vi "niDTS WLAN UTIL to Type.vi"(4 "N_SS":i32=1, 6 "MCS":i32, 9 "OFDM Data Rate (Mbps)":T1, 10 "DSSS Data Rate (Mbps)":T2, 11 "Standard":T3 caption="802.11 Standard") -> (2 "WLAN Type":T4)   [LabVIEW 2015, in "niDTS WLAN.lvlib"]
uses:
  niDTS WLAN.lvlib
  Includes/niDTS WLAN INC Type.ctl
  Includes/niDTS WLAN INC Standard.ctl
  Includes/niDTS WLAN INC DSSS Data Rate.ctl
  Includes/niDTS WLAN INC OFDM Data Rate.ctl
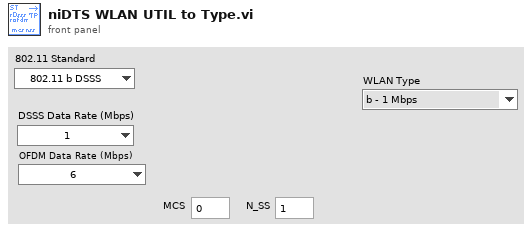
[diagram p1: front panel]
types:
  T1 = typedef "niDTS WLAN.lvlib/niDTS WLAN INC OFDM Data Rate.ctl" = enum16{"6", "9", "12", "18", "24", "36", "48", "54"}
  T2 = typedef "niDTS WLAN.lvlib/niDTS WLAN INC DSSS Data Rate.ctl" = enum16{"1", "2", "5.5", "11"}
  T3 = typedef "niDTS WLAN.lvlib/niDTS WLAN INC Standard.ctl" = enum16{"802.11 b DSSS", "802.11 a/g OFDM", "802.11 n HT", "802.11 ac VHT"}
  T4 = typedef "niDTS WLAN.lvlib/niDTS WLAN INC Type.ctl" = enum16{"b - 1 Mbps", "b - 2 Mbps", "b - 5.5 Mbps", "b - 11 Mbps", "ag - 6 Mbps", "ag - 9 Mbps", "ag - 12 Mbps", "ag - 18 Mbps", "ag - 24 Mbps", "ag - 36 Mbps", "ag - 48 Mbps", "ag - 54 Mbps", "n - MCS0", "n - MCS1", "n - MCS2", "n - MCS3", "n - MCS4", "n - MCS5", "n - MCS6", "n - MCS7", "n - MCS8", "n - MCS9", "n - MCS10", "n - MCS11", "n - MCS12", "n - MCS13", "n - MCS14", "n - MCS15", "n - MCS16", "n - MCS17", "n - MCS18", "n - MCS19", "n - MCS20", "n - MCS21", "n - MCS22", "n - MCS23", "n - MCS24", "n - MCS25", "n - MCS26", "n - MCS27", "n - MCS28", "n - MCS29", "n - MCS30", "n - MCS31", "ac - MCS0 -1", "ac - MCS1 -1", "ac - MCS2 -1", "ac - MCS3 -1", "ac - MCS4 -1", "ac - MCS5 -1", "ac - MCS6 -1", "ac - MCS7 -1", "ac - MCS8 -1", "ac - MCS9 -1", "ac - MCS0 -2", "ac - MCS1 -2", "ac - MCS2 -2", "ac - MCS3 -2", "ac - MCS4 -2", "ac - MCS5 -2", "ac - MCS6 -2", "ac - MCS7 -2", "ac - MCS8 -2", "ac - MCS9 -2", "ac - MCS0 -3", "ac - MCS1 -3", "ac - MCS2 -3", "ac - MCS3 -3", "ac - MCS4 -3", "ac - MCS5 -3", "ac - MCS6 -3", "ac - MCS7 -3", "ac - MCS8 -3", "ac - MCS9 -3", "ac - MCS0 -4", "ac - MCS1 -4", "ac - MCS2 -4", "ac - MCS3 -4", "ac - MCS4 -4", "ac - MCS5 -4", "ac - MCS6 -4", "ac - MCS7 -4", "ac - MCS8 -4", "ac - MCS9 -4"}
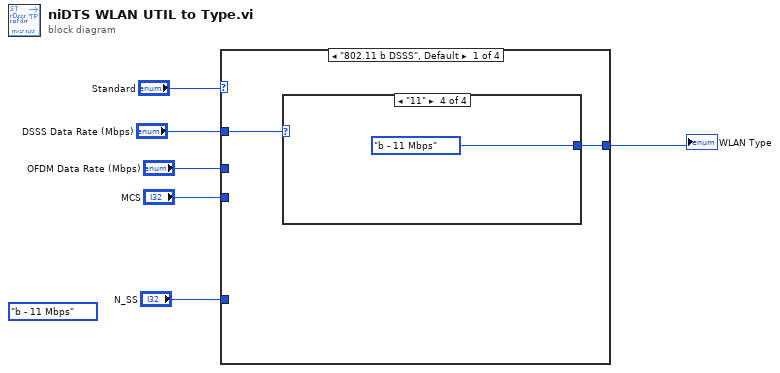
[diagram p0: block diagram]
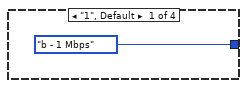
[diagram p2: hidden frame]
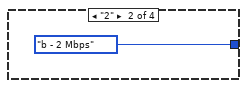
[diagram p3: hidden frame]
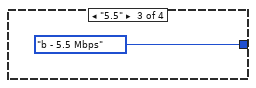
[diagram p4: hidden frame]
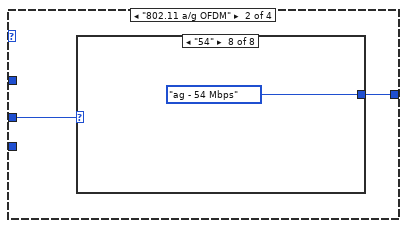
[diagram p5: hidden frame]
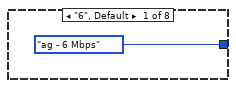
[diagram p6: hidden frame]
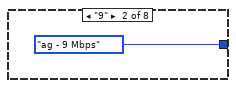
[diagram p7: hidden frame]
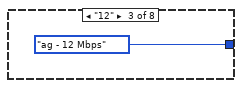
[diagram p8: hidden frame]
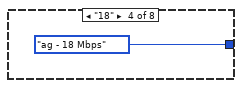
[diagram p9: hidden frame]
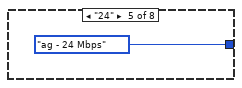
[diagram p10: hidden frame]
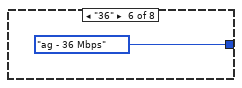
[diagram p11: hidden frame]
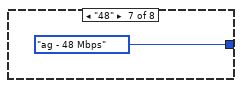
[diagram p12: hidden frame]
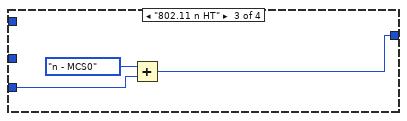
[diagram p13: hidden frame]
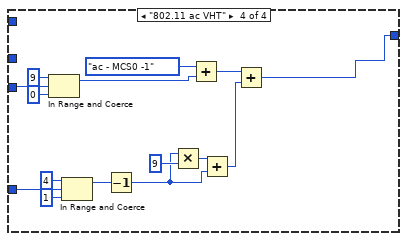
[diagram p14: hidden frame]
diagram:
  (unwired) niDTS_WLAN_INC_Type."b - 11 Mbps" ("WLAN Type")
  n1 = case shown="\"802.11 b DSSS\", Default" "Standard" {
    tunnel: "DSSS Data Rate (Mbps)" -> [w8 _ _ _]
    tunnel: [w7 w13 w23 w37] -> w4
    tunnel: "OFDM Data Rate (Mbps)" -> [_ w14 _ _]
    tunnel: "MCS" -> [_ _ w24 w36]
    tunnel: "N_SS" -> [_ _ _ w30]
    frame "802.11 b DSSS", Default {
      n2 = case shown="\"11\"" w8 {
        tunnel: [niDTS_WLAN_INC_Type."b - 1 Mbps" ("WLAN Type") niDTS_WLAN_INC_Type."b - 2 Mbps" ("WLAN Type") niDTS_WLAN_INC_Type."b - 5.5 Mbps" ("WLAN Type") niDTS_WLAN_INC_Type."b - 11 Mbps" ("WLAN Type")] -> w7
        frame "1", Default {
        }
        frame "2" {
        }
        frame "5.5" {
        }
        frame "11" {
        }
      }
    }
    frame "802.11 a/g OFDM" {
      n3 = case shown="\"54\"" w14 {
        tunnel: [niDTS_WLAN_INC_Type."ag - 6 Mbps" ("WLAN Type") niDTS_WLAN_INC_Type."ag - 9 Mbps" ("WLAN Type") niDTS_WLAN_INC_Type."ag - 12 Mbps" ("WLAN Type") niDTS_WLAN_INC_Type."ag - 18 Mbps" ("WLAN Type") niDTS_WLAN_INC_Type."ag - 24 Mbps" ("WLAN Type") niDTS_WLAN_INC_Type."ag - 36 Mbps" ("WLAN Type") niDTS_WLAN_INC_Type."ag - 48 Mbps" ("WLAN Type") niDTS_WLAN_INC_Type."ag - 54 Mbps" ("WLAN Type")] -> w13
        frame "6", Default {
        }
        frame "9" {
        }
        frame "12" {
        }
        frame "18" {
        }
        frame "24" {
        }
        frame "36" {
        }
        frame "48" {
        }
        frame "54" {
        }
      }
    }
    frame "802.11 n HT" {
      n4 = Add(x=niDTS_WLAN_INC_Type."n - MCS0" ("WLAN Type"), y=w24) -> (x+y=w23:i32)
    }
    frame "802.11 ac VHT" {
      n5 = In Range and Coerce(upper limit=9, x=w36, lower limit=0) -> (coerced(x)=w33:i32)  [unwired: 1 out]
      n6 = In Range and Coerce(upper limit=4, x=w30, lower limit=1) -> (coerced(x)=w29:i32)  [unwired: 1 out]
      n7 = Decrement(x=w29) -> (x-1=w27:i32)
      n8 = Multiply(x=w27, y=9) -> (x*y=w28:i32)
      n9 = Add(x=niDTS_WLAN_INC_Type."ac - MCS0 -1" ("WLAN Type"), y=w33) -> (x+y=w39:i32)
      n10 = Add(x=w28, y=w27) -> (x+y=w26:i32)
      n11 = Add(x=w39, y=w26) -> (x+y=w37:i32)
    }
  }
  "WLAN Type" <- w4
